vi "Periodic State String.vi"(4 "Do State Now? (Reset Period)":bool, 6 "Period (ms)":u32, 9 "State":string) -> (1 "State Out":string)   [LabVIEW 2013]
doc: "Periodically passes the <b>State</b> string though the function at intervals defined by <b>Period (ms)</b> or when first called.\nThe <b>State</b> string can also be passed through immediately when <b>Do State Now? (Reset Period)</b> is TRUE.\n\nFor instructions on how to use the JKI State Machine, examples and video tutorials, visit:\nhttp://jkisoft.com/state-machine/"
panel:
  # "For instructions on how to use the JKI State Machine, examples and video tutorials, visit:\nhttp://jki.net/state-machine/\n\nJKI State Machine™\nhttp://jki.net/state-machine/\nCopyright (C) 2005-2024, JKI <info@jki.net>\nALL RIGHTS RESERVED"
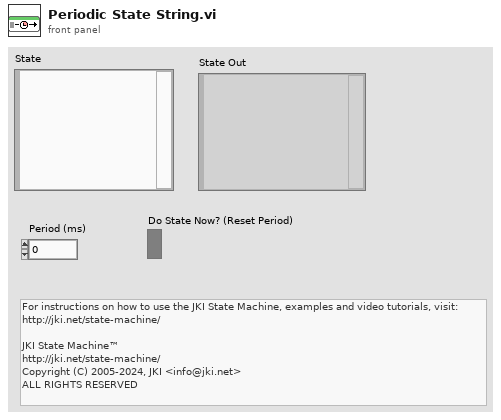
[diagram p1: front panel]
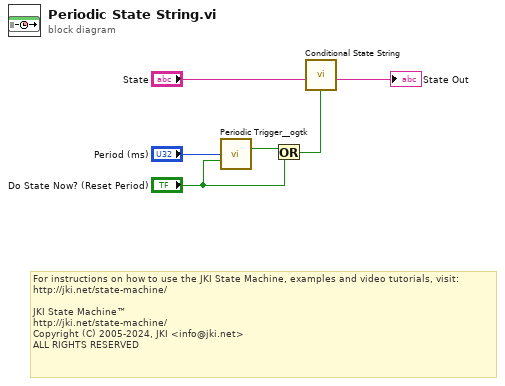
[diagram p0: block diagram]
diagram:
  # "For instructions on how to use the JKI State Machine, examples and video tutorials, visit:\nhttp://jki.net/state-machine/\n\nJKI State Machine™\nhttp://jki.net/state-machine/\nCopyright (C) 2005-2024, JKI <info@jki.net>\nALL RIGHTS RESERVED"
  n1 = call <userlib>:"Periodic Trigger__ogtk.vi"("time (ms)"="Period (ms)", "reset"="Do State Now? (Reset Period)") -> ("Triggered"=w2:bool)  [unwired: 11 in, 2 out]
  n2 = Or(x=w2, y="Do State Now? (Reset Period)") -> (x .or. y?=w1:bool)
  n3 = call "Conditional State String.vi"("Do State(s)?"=w1, "State"="State") -> ("State Out"=→"State Out":string)  [unwired: 7 in]
